vi "GraphicUI.events.get.vi"(11 "manager_daemon in":refnum<class "manager_daemon.lvclass">) -> (2 "graphic ui events":T1, 3 "manager_daemon out":refnum<class "manager_daemon.lvclass">)   [LabVIEW 2024, in "manager_daemon.lvclass"]
uses:
  manager_daemon.lvclass
  manager_daemon.lvclass/manager_daemon.ctl
  CV_Shared_Library/volume.type--enum.ctl
  CV_Shared_Library/CV_Shared_Library.lvlib
  TypeDefs/issue.display--cluster.ctl
  CV_Shared_Library/volume.object--cluster.ctl
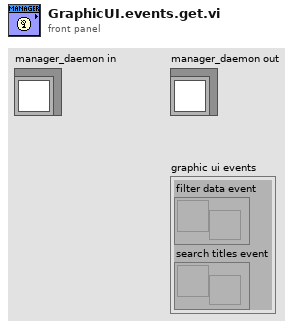
[diagram p1: front panel]
types:
  T1 = cluster{"filter data event":refnum<user-event>, "search titles event":refnum<user-event>}
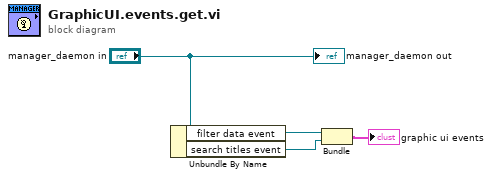
[diagram p0: block diagram]
diagram:
  n1 = Unbundle By Name("manager_daemon in") -> ("filter data event"=w3:refnum<user-event>, "search titles event"=w2:refnum<user-event>)
  n2 = Bundle("filter data event"=w3, "search titles event"=w2) -> (→"graphic ui events":T1)  [unwired: 1 in]
  "manager_daemon out" <- "manager_daemon in"
